vi "test_joystick2.vi"() -> ()   [LabVIEW 2021]
uses:
  Ctrl/joystick cfg.ctl
  Ctrl/joy-axis.ctl
  Ctrl/cmd_common.ctl
panel:
  in  "Joystick cfg 2":T1={"steer limit"={"scale"=10.0, "offset"=42.0}, "speed limit"={"min"=10.0, "max"=42.0}, "Axis"={"man"=0.0, "auto"=0.0, "angular"=enum."X axis", "linear"=enum."Z rotation", "linear inv"=FALSE, "ang inv"=FALSE}} {"speed limit"."max" min=0.0 max=254.0 step=1.0}
  out "default val check":bool
  in  "stop":bool
  out "Cluster":cluster{dbl, dbl} {"?" format="%#.1f"; "?" format="%.1f"}
  out "n":i32=34
  out "XY Graph":cluster{cluster{"X":dbl, "Y":dbl}[]}[](graph)
  # "RLCar Joystick contol sw"
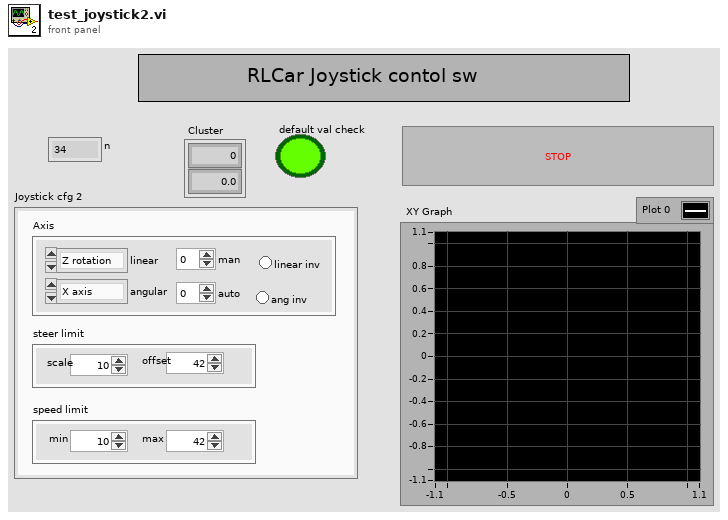
[diagram p1: front panel]
types:
  T1 = typedef "joystick cfg.ctl" = cluster{"steer limit":cluster{"scale":dbl, "offset":dbl}, "speed limit":cluster{"min":dbl, "max":dbl}, "Axis":cluster{"man":dbl, "auto":dbl, "angular":T2, "linear":T2, "linear inv":bool, "ang inv":bool}}
  T2 = typedef "joy-axis.ctl" = enum16{"X axis", "Y axis", "Z axis", "X rotation", "Y rotation", "Z rotation", "U axis", "V axis"}
  T3 = cluster{"axis info":cluster{"X axis":i32, "Y axis":i32, "Z axis":i32, "X axis rotation":i32, "Y axis rotation":i32, "Z axis rotation":i32, "U axis":i32, "V axis":i32}, "button info":cluster{"button 1":bool, "button 2":bool, "button 3":bool, "button 4":bool, "button 5":bool, "button 6":bool, "button 7":bool, "button 8":bool, "button 9":bool, "button 10":bool, "button 11":bool, "button 12":bool, "button 13":bool, "button 14":bool, "button 15":bool, "button 16":bool, "button 17":bool, "button 18":bool, "button 19":bool, "button 20":bool, "button 21":bool, "button 22":bool, "button 23":bool, "button 24":bool, "button 25":bool, "button 26":bool, "button 27":bool, "button 28":bool, "button 29":bool, "button 30":bool, "button 31":bool, "button 32":bool}, "direction info":cluster{"pov 1":i32, "pov 2":i32, "pov 3":i32, "pov 4":i32}}
  T4 = typedef "cmd_common.ctl" = enum16{"read", "write"}
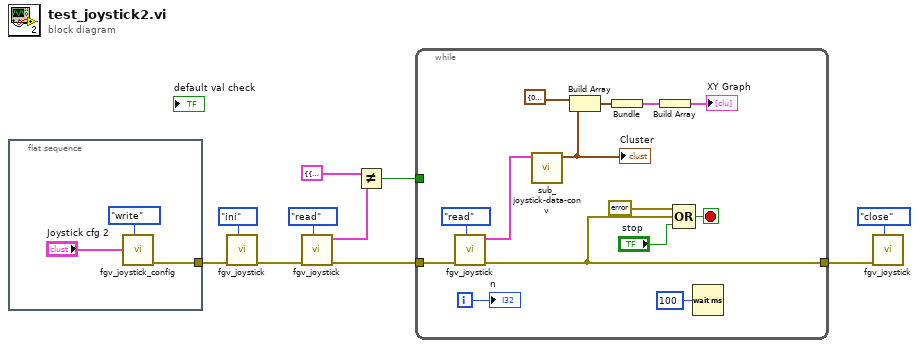
[diagram p0: block diagram]
diagram:
  n1 = flat-sequence {
    tunnel: [w12] -> w1
    frame #0 {
      n2 = call "fgv_joystick_config.vi"("cmd"=cmd_common."write", "Joystick cfg 2"="Joystick cfg 2") -> ("error out"=w12:errorcluster)  [unwired: 8 in, 1 out]
    }
  }
  n3 = call "fgv_joystick.vi"("cmd"=enum16{"ini", "read", "close"}."ini", "error in"=w1) -> ("error out"=w6:errorcluster)  [unwired: 7 in, 2 out]
  n4 = call "fgv_joystick.vi"("cmd"=enum16{"ini", "read", "close"}."read", "error in"=w6) -> ("error out"=w5:errorcluster, "joystick info-out"=w3:T3)  [unwired: 7 in, 1 out]
  n5 = Not Equal?(x=T3 {"axis info"={"X axis"=0, "Y axis"=-256, "Z axis"=0, "X axis rotation"=0, "Y axis rotation"=0, "Z axis rotation"=-256, "U axis"=0, "V axis"=0}, "button info"={"button 1"=FALSE, "button 2"=FALSE, "button 3"=FALSE, "button 4"=FALSE, "button 5"=FALSE, "button 6"=FALSE, "button 7"=FALSE, "button 8"=FALSE, "button 9"=FALSE, "button 10"=FALSE, "button 11"=FALSE, "button 12"=FALSE, "button 13"=FALSE, "button 14"=FALSE, "button 15"=FALSE, "button 16"=FALSE, "button 17"=FALSE, "button 18"=FALSE, "button 19"=FALSE, "button 20"=FALSE, "button 21"=FALSE, "button 22"=FALSE, "button 23"=FALSE, "button 24"=FALSE, "button 25"=FALSE, "button 26"=FALSE, "button 27"=FALSE, "button 28"=FALSE, "button 29"=FALSE, "button 30"=FALSE, "button 31"=FALSE, "button 32"=FALSE}, "direction info"={"pov 1"=-1, "pov 2"=-1, "pov 3"=-1, "pov 4"=-1}} ("joystick info-out 2"), y=w3) -> (x != y?=w2:bool)
  n6 = while {
    tunnel: [w24] -> w8
    tunnel: w5 -> [w25]
    tunnel: w2 -> [_]
    i -> [w21]
    stop <- w22 stop-if-true
    n7 = call "fgv_joystick.vi"("cmd"=enum16{"ini", "read", "close"}."read", "error in"=w25) -> ("error out"=w24:errorcluster, "joystick info-out"=w15:T3)  [unwired: 7 in, 1 out]
    n8 = call "sub_joystick-data-conv.vi"("joystick info-in"=w15) -> ("opval"=w14:cluster{dbl, dbl})  [unwired: 9 in, 1 out]
    "Cluster" <- w14
    n9 = Build Array(cluster{"X":dbl, "Y":dbl} {"X"=0.0, "Y"=0.0}, w14) -> (w19:cluster{"X":dbl, "Y":dbl}[])
    n10 = Bundle(w19) -> (w18:cluster{cluster{"X":dbl, "Y":dbl}[]})  [unwired: 1 in]
    n11 = Build Array(w18) -> (→"XY Graph":cluster{cluster{"X":dbl, "Y":dbl}[]}[])
    n12 = Compound Arithmetic op=OR(errorcluster {"status"=FALSE, "code"=0, "source"=""} ("value"), w24, "stop") -> (w22:bool)
    n13 = Wait (ms)(milliseconds to wait=u32 100) -> ()  [unwired: 1 out]
    "n" <- w21
  }
  n14 = call "fgv_joystick.vi"("cmd"=enum16{"ini", "read", "close"}."close", "error in"=w8) -> ()  [unwired: 7 in, 3 out]
